vi "pathrun.vi"() -> (2 "引用句柄输出":refnum<file>)   [LabVIEW 2018]
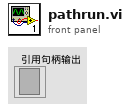
[diagram p1: front panel]
types:
  T1 = enum16{"open", "replace", "create", "open or create", "replace or create", "replace or create with confirmation"}
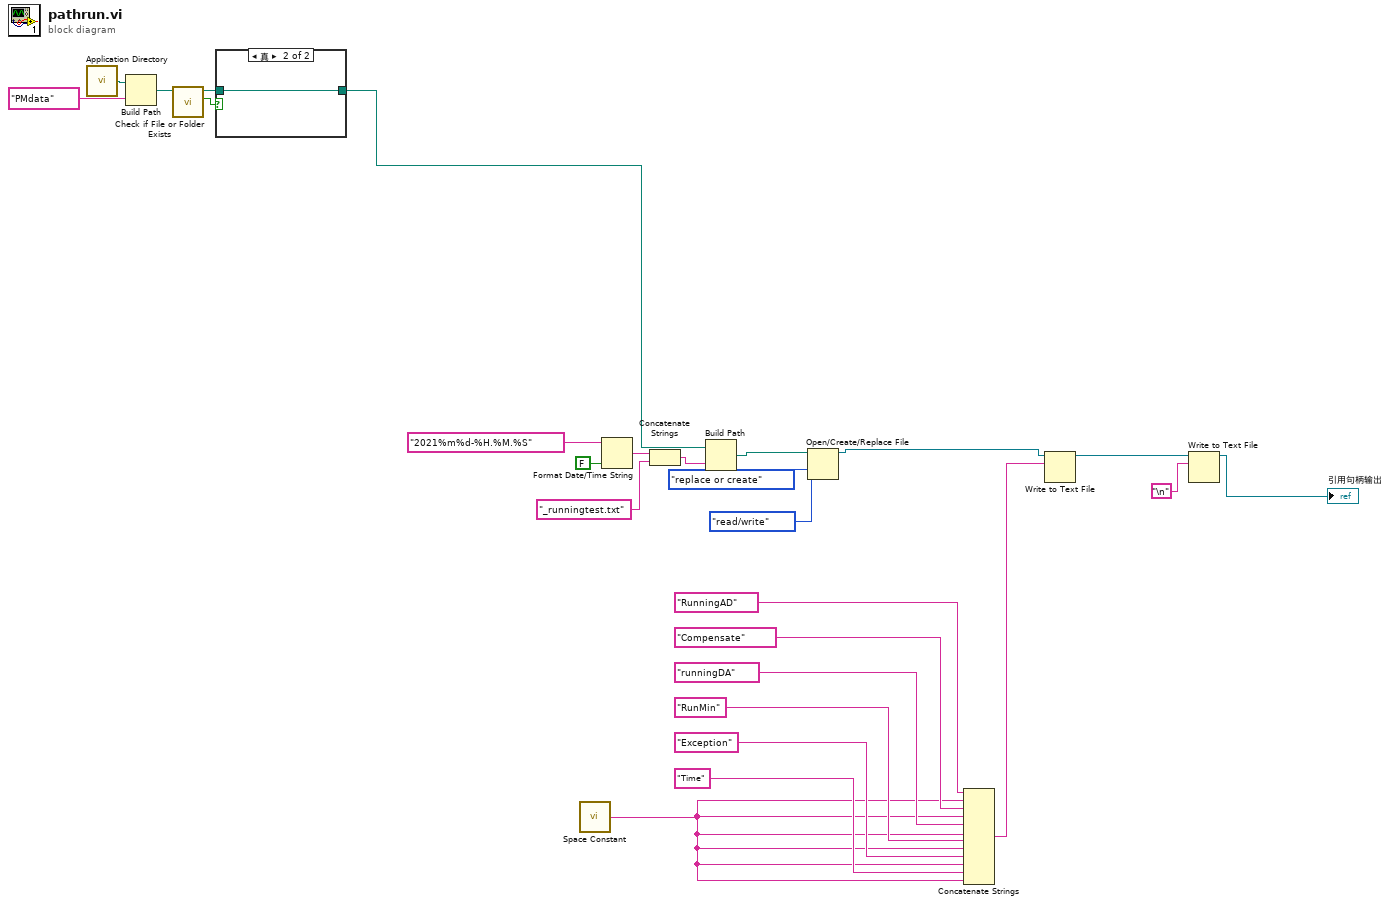
[diagram p0: block diagram]
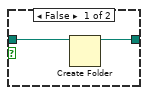
[diagram p2: hidden frame]
diagram:
  n1 = call <vilib>:"Application Directory.vi"() -> ("Application Directory"=w26:path)
  n2 = Build Path(base path=w26, name or relative path="PMdata" ("时间格式字符串(%c)")) -> (appended path=w24:path)
  n3 = call <vilib>:"Check if File or Folder Exists.vi"("path"=w24) -> ("file or folder exists?"=w23:bool, "dup path"=w22:path)  [unwired: 8 in, 1 out]
  n4 = case shown="真" w23 {
    tunnel: [w27 w29] -> w15
    tunnel: w22 -> [w28 w29]
    frame False {
      n5 = Create Folder(path (use dialog)=w28) -> (created path=w27:path)  [unwired: 2 in, 2 out]
    }
    frame True {
    }
  }
  n6 = call <vilib>:"Space Constant.vi"() -> ("String"=w1:string)
  n7 = Format Date/Time String(time format string (%c)="2021%m%d-%H.%M.%S" ("时间格式字符串(%c)"), UTC format=FALSE ("UTC格式")) -> (date/time string=w19:string)  [unwired: 1 in]
  n8 = Concatenate Strings(w19, "_runningtest.txt" ("字符串")) -> (w17:string)
  n9 = Build Path(base path=w15, name or relative path=w17) -> (appended path=w21:path)
  n10 = Open/Create/Replace File(file path (use dialog)=w21, operation (0:open)=T1."replace or create" ("操作(0:open)"), access (0:read/write)=enum16{"read/write", "read-only", "write-only"}."read/write" ("权限(0:read/write)")) -> (refnum out=w4:refnum<file>)  [unwired: 3 in, 2 out]
  n11 = Concatenate Strings("RunningAD" ("字符串"), w1, "Compensate" ("字符串"), w1, "runningDA" ("字符串"), w1, "RunMin" ("字符串"), w1, "Exception" ("字符串"), w1, "Time" ("字符串"), w1) -> (w5:string)
  n12 = Write to Text File ("写入文本文件")(file (use dialog)=w4, text=w5) -> (refnum out=w11:refnum<file>)  [unwired: 2 in, 2 out]
  n13 = Write to Text File(file (use dialog)=w11, text="\n") -> (refnum out=→"引用句柄输出":refnum<file>)  [unwired: 2 in, 2 out]
